vi "模式一 - 副本.vi"(0 "Input Handle":cluster{"Session":u32, "Card number":u32}, 1 "接收端数量":i32, 2 "文件类型":u16(ring) items=["txt", "xls", "cvs", "xlsx"], 3 "接收端":i32=1 min=1 max=64 step=1, 5 "激励端":i32=1 min=1 max=64 step=1, 7 "VISA 资源":refnum<visa-resource-name>, 9 "t2":u32, 10 "t1":u32, 11 "error in":errorcluster {"code" format="%.0x"}, 12 "起始点数":i32, 13 "终止点数":i32, 14 "t4":u32) -> (4 "Output Handle":cluster{"Session":u32, "Card number":u32}, 15 "error out":errorcluster caption="error in")   [LabVIEW 2018]
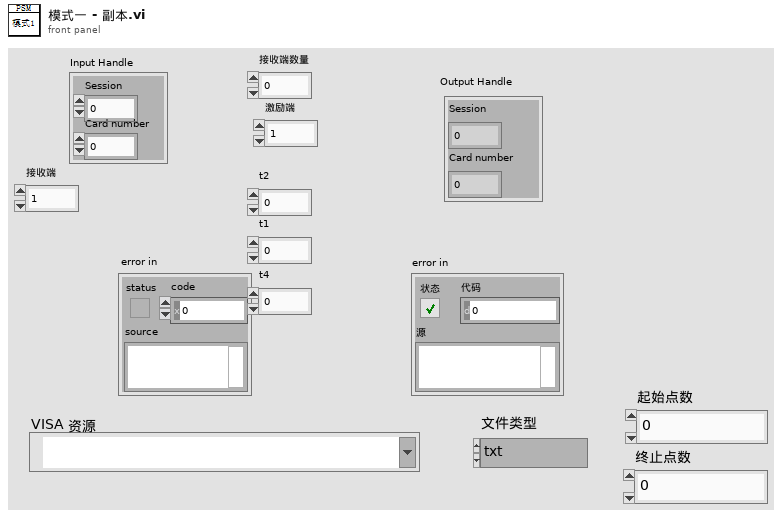
[diagram p1: front panel]
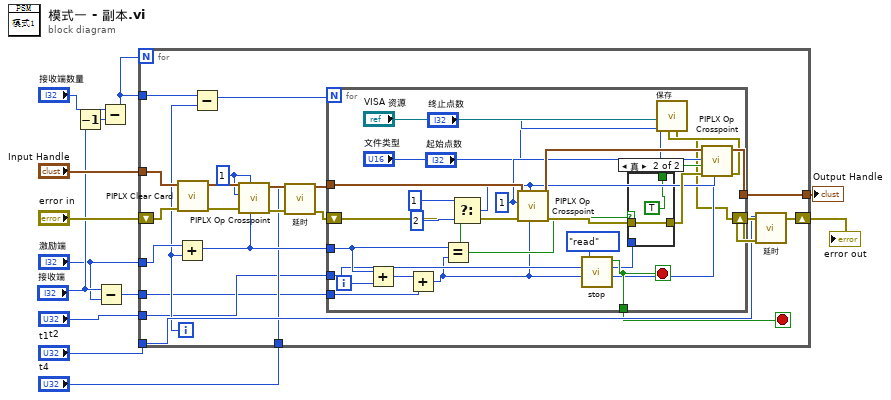
[diagram p0: block diagram]
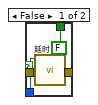
[diagram p2: hidden frame]
diagram:
  n1 = Decrement(x="接收端") -> (x-1=w5:i32)
  n2 = Subtract(x="接收端", y="激励端") -> (x-y=w1:i32)
  n3 = Subtract(x="接收端数量", y=w5) -> (x-y=w4:i32)
  n4 = for {
    N: w4 -> [_]
    tunnel: "激励端" -> [w30]
    tunnel: "Input Handle" -> [w28]
    tunnel: "t2" -> [w16]
    shift-right: [w32] -> w9
    shift-left: "error in" -> [w27]
    tunnel: [w34] -> w10
    tunnel: "t1" -> [w31]
    tunnel: "t4" -> [w17]
    tunnel: w1 -> [w15]
    tunnel: w4 -> [w14]
    i -> [w26]
    stop <- w29 stop-if-true
    w21 = u32 1 ("Row")
    n5 = Add(x=w30, y=w26) -> (x+y=w20:i32)
    n6 = call <instrlib>:"PIPLX Clear Card.vi"("error in"=w27, "Input Handle"=w28) -> ("error out"=w24:errorcluster, "Output Handle"=w23:cluster{"Session":u32, "Card number":u32})  [unwired: 8 in]
    n7 = Subtract(x=w14, y=w26) -> (x-y=w25:i32)
    n8 = call <instrlib>:"PIPLX Op Crosspoint.vi"("Column"=w20, "Row"=w21, "error in"=w24, "Output Subunit"=w21, "Input Handle"=w23) -> ("error out"=w19:errorcluster, "Output Handle"=w22:cluster{"Session":u32, "Card number":u32})  [unwired: 5 in]
    n9 = call "延时.vi"("error in (no error)"=w19, "延时（百毫秒）"=w17) -> ("error out"=w18:errorcluster)  [unwired: 9 in]
    n10 = for {
      N: w25 -> [_]
      tunnel: w20 -> [w57]
      tunnel: w22 -> [w56]
      tunnel: w16 -> [w51]
      shift-right: [w35] -> w33
      shift-left: w18 -> [w55]
      tunnel: [w49] -> w34
      tunnel: [w53] -> w29
      tunnel: w15 -> [w43]
      i -> [w60]
      stop <- w53 stop-if-true
      w46 = u32 1 ("Output Subunit")
      n11 = Add(x=w57, y=w60) -> (x+y=w44:i32)
      n12 = Add(x=w44, y=w43) -> (x+y=w42:i32)
      n13 = Equal?(x=w57, y=w42) -> (x = y?=w50:bool)
      n14 = Select(t=u32 1 ("Row"), s=w50, f=u32 2) -> (s? t:f=w45:u32)
      n15 = call <instrlib>:"PIPLX Op Crosspoint.vi"("Column"=w42, "Row"=w45, "error in"=w55, "Output Subunit"=w46, "Input Handle"=w56) -> ("error out"=w54:errorcluster, "Output Handle"=w48:cluster{"Session":u32, "Card number":u32})  [unwired: 5 in]
      n16 = call "stop.vi"("枚举"=enum16{"write", "read"}."read") -> ("停止"=w53:bool)  [unwired: 10 in]
      n17 = case shown="真" w50 {
        tunnel: w54 -> [w64 w66]
        tunnel: [w63 w66] -> w47
        tunnel: w51 -> [w62 _]
        tunnel: [FALSE ("Action") TRUE ("Action")] -> w41
        frame False {
          n18 = call "延时.vi"("error in (no error)"=w64, "延时（百毫秒）"=w62) -> ("error out"=w63:errorcluster)  [unwired: 9 in]
        }
        frame True {
        }
      }
      n19 = call <instrlib>:"PIPLX Op Crosspoint.vi"("Column"=w42, "Row"=w45, "error in"=w47, "Action"=w41, "Output Subunit"=w46, "Input Handle"=w48) -> ("error out"=w36:errorcluster, "Output Handle"=w49:cluster{"Session":u32, "Card number":u32})  [unwired: 4 in]
      n20 = call "保存.vi"("error in (no error)"=w36, "终止点数"="终止点数", "起始点数"="起始点数", "文件类型"="文件类型", "VISA 资源"="VISA 资源") -> ("error out"=w35:errorcluster)  [unwired: 6 in]
    }
    n21 = call "延时.vi"("error in (no error)"=w33, "延时（百毫秒）"=w31) -> ("error out"=w32:errorcluster)  [unwired: 9 in]
  }
  "Output Handle" <- w10
  "error out" <- w9
